vi "PH_PP_CurrentMeas.panel.vi"(0 "object ref":refnum<vi>, 5 "error in (no error)":errorcluster) -> (19 "error out":errorcluster)   [LabVIEW 2014, in "PH_PP_CurrentMeas.lvlib"]
doc: "This is just an example for a GUI thread.\n\nLicense Agreement for this software:\n\nCopyright (C)\nGesellschaft für Schwerionenforschung, GSI\nPlanckstr. 1\n64291 Darmstadt\nGermany\n\nContact: D.Beck@gsi.de \n\nThis program is free software; you can redistribute it and/or modify it under the terms of the GNU General Public License as published by the Free Software Foundation; either version 2 of the license, or (at your option) any later version.\n\nThis program is distributed in the hope that it will be useful, but WITHOUT ANYW ARRANTY; without even the implied warranty of MERCHANTABILITY or FITNESS FOR A PARTICULAR PURPOSE. See the GNU General License for more details (http://www.gnu.org).\n\nGesellschaft für Schwerionenforschung, GSI\nPlanckstr. 1, 64291 Darmstadt, Germany\nFor all questions and ideas contact: M.Richter@gsi.de, H.Brand@gsi.de or D.Beck@gsi.de.\nLast update: 18-DEC-2002"
uses:
  PH_PP_CurrentMeas.lvlib
  PH_Basics/PH_StatusHandler/PH_StatusHandler.GUI element.ctl
  PH_PP_CurrentMeas.CommandCluster.ctl
  CS_Core/CSObj/CSObj.lvlib
  PH_Basics/PH_Common/PH_Common.lvlib
  PH_Basics/PH_Class/PH_Class.lvlib
  PH_Basics/PH_PSDBWriter/PH_PSDBWriter.lvlib
  PH_Basics/PH_StatusHandler/PH_StatusHandler.lvlib
panel:
  in  "Start Task 3":bool
  in  "Start Task 2":bool
  in  "Start Task 1":bool
  out "Task FR and PPPA Bar":u32(colorbox) caption="Powermeter"
  out "Task PPMA FR and PPPA":u32(colorbox) caption="PPMA FR and PPPA"
  out "Task PPMA PU 3 ... 5 Bar":u32(colorbox) caption="Powermeter"
  out "Task PPMA PU 3 ... 5":u32(colorbox) caption="PPMA PU 3 ... 5"
  out "Task PPMA PU 1 ... 3 Bar":u32(colorbox) caption="Powermeter"
  out "Task PPMA PU 1 ... 3":u32(colorbox) caption="PPMA PU 1 ... 3"
  out "Sequencer State":string
  out "PSDB Status":u32(colorbox)=6618880 caption="PSDB"
  out "Status":T1 caption="Enabling State"
  in  "Exit":bool
  in  "stop":bool
  in  "Tab Control":T2(tab)
  out "PreAmp Data":waveform(dbl)[](graph) caption="Measurement data"
  out "Status 45mm":T1 caption="45mm"
  out "Status 19mm - 2":T1 caption="19mm - 2"
  out "Status 19mm - 1":T1 caption="19mm - 1"
  out "Data PU 1":waveform(dbl)[](graph) caption="Measurement data"
  out "Status PU1":T1 caption="Enabling State"
  out "Data PU 2":waveform(dbl)[](graph) caption="Measurement data"
  out "Status PU2":T1 caption="Enabling State"
  out "Data PU 3":waveform(dbl)[](graph) caption="Measurement data"
  out "Status PU3":T1 caption="Enabling State"
  out "Data PU 4":waveform(dbl)[](graph) caption="Measurement data"
  out "Status PU4":T1 caption="Enabling State"
  out "Data PU 5":waveform(dbl)[](graph) caption="Measurement data"
  out "Status PU5":T1 caption="Enabling State"
  out "Data PU FR":waveform(dbl)[](graph) caption="Measurement data"
  out "Status FR":T1 caption="Enabling State"
  out "Hardware Feedback":T4(array[cluster])
  # "PCS"
  # "3.40"
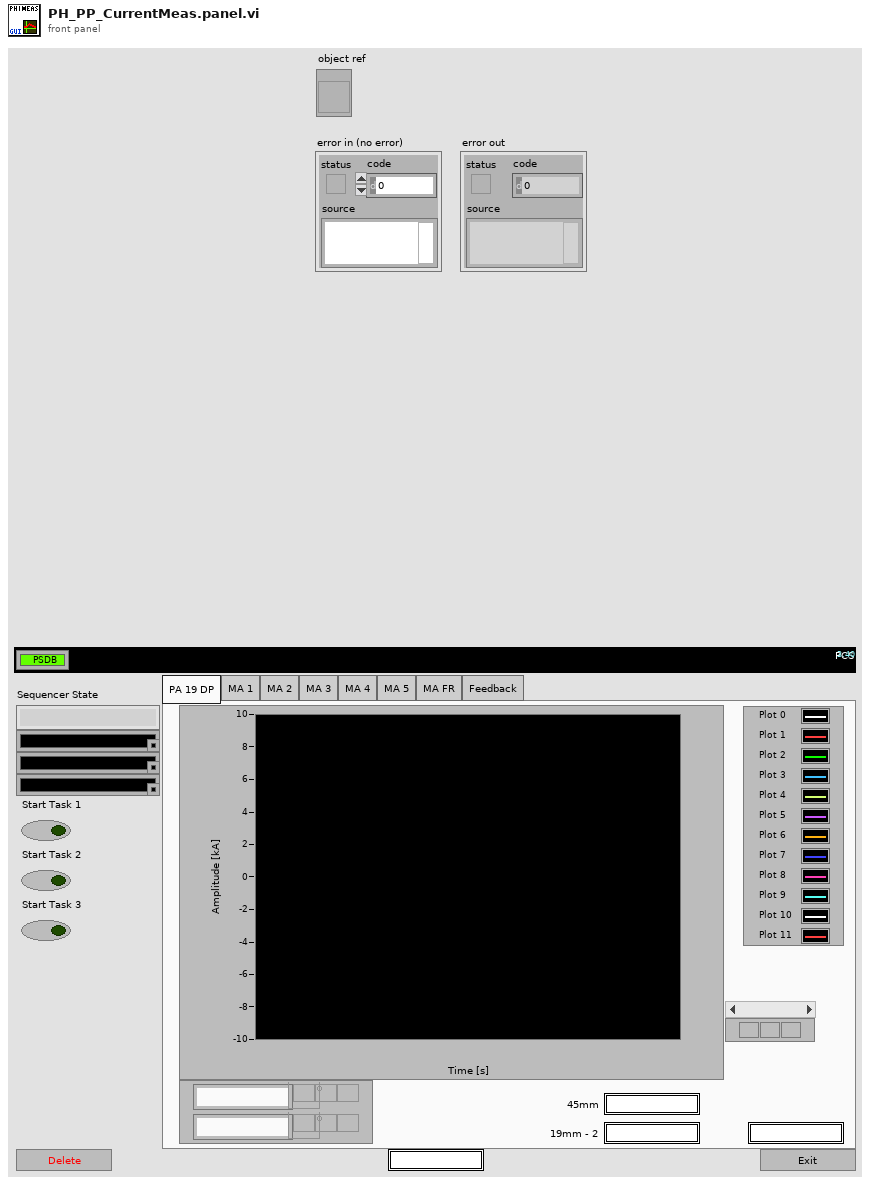
[diagram p1: front panel]
types:
  T1 = typedef "PH_StatusHandler.lvlib/PH_StatusHandler.GUI element.ctl" = u16
  T2 = enum32{"PA 19 DP", "MA 1", "MA 2", "MA 3", "MA 4", "MA 5", "MA FR", "Feedback"}
  T3 = typedef "PH_PP_CurrentMeas.lvlib/PH_PP_CurrentMeas.CommandCluster.ctl" = cluster{"Command":string, "Data":string, "error out":errorcluster}
  T4 = cluster{"Received Data Sets":T3[], "Driver Error":errorcluster, "Connection not established":bool, "Error unpacking the data":bool, "No Task defined":bool, "Not triggered yet":bool}[]
  T5 = typedef "PH_PP_CurrentMeas.lvlib/PH_PP_CurrentMeas.i attribute.ctl" = cluster{"Status":cluster{"GUI Ref Hardware Feedback":refnum<vi>, "Tab Control":refnum<vi>}, "PU 1":cluster{"Instance":string, "Status":T6, "Ref Status ":refnum<vi>, "Data":waveform(dbl)[], "Ref Data":refnum<vi>}, "PU 2":cluster{"Instance":string, "Status":T6, "Ref Status ":refnum<vi>, "Data":waveform(dbl)[], "Ref Data":refnum<vi>}, "PU 3":cluster{"Instance":string, "Status":T6, "Ref Status ":refnum<vi>, "Data":waveform(dbl)[], "Ref Data":refnum<vi>}, "PU 4":cluster{"Instance":string, "Status":T6, "Ref Status ":refnum<vi>, "Data":waveform(dbl)[], "Ref Data":refnum<vi>}, "PU 5":cluster{"Instance":string, "Status":T6, "Ref Status ":refnum<vi>, "Data":waveform(dbl)[], "Ref Data":refnum<vi>}, "FR":cluster{"Instance":string, "Status":T6, "Ref Status ":refnum<vi>, "Data":waveform(dbl)[], "Ref Data":refnum<vi>}, "PA - 19mm 1":cluster{"Instance":string, "Status":T6, "Ref Status ":refnum<vi>}, "PA - 19mm 2":cluster{"Instance":string, "Status":T6, "Ref Status ":refnum<vi>, "no link":bool}, "PA - 45mm":cluster{"Instance":string, "Status":T6, "Ref Status ":refnum<vi>, "no link":bool}, "PA Data":cluster{"Data":waveform(dbl)[], "Ref":refnum<vi>}, "Sequencer":cluster{"Instance":string, "SM State Ref":refnum<vi>}, "Tasks":cluster{"Port":u16, "connection ID":refnum<k5>, "Status":T6, "Ref":refnum<vi>, "Ref Bar":refnum<vi>, "Feedback":cluster{"Received Data Sets":T3[], "Driver Error":errorcluster, "Connection not established":bool, "Error unpacking the data":bool, "No Task defined":bool, "Not triggered yet":bool}, "Data":waveform(dbl)[], "Ref Teststart Task":refnum<vi>}[], "in use":cluster{"MA DP":bool, "FR and PA":bool}, "DAQ Server":string}
  T6 = typedef "PH_StatusHandler.lvlib/PH_StatusHandler.Status.ctl" = i16
  T7 = cluster{"Port":u16, "connection ID":refnum<k5>, "Status":T6, "Ref":refnum<vi>, "Ref Bar":refnum<vi>, "Feedback":cluster{"Received Data Sets":T3[], "Driver Error":errorcluster, "Connection not established":bool, "Error unpacking the data":bool, "No Task defined":bool, "Not triggered yet":bool}, "Data":waveform(dbl)[], "Ref Teststart Task":refnum<vi>}[]
  T8 = cluster{"Port":u16, "connection ID":refnum<k5>, "Status":T6, "Ref":refnum<vi>, "Ref Bar":refnum<vi>, "Feedback":cluster{"Received Data Sets":T3[], "Driver Error":errorcluster, "Connection not established":bool, "Error unpacking the data":bool, "No Task defined":bool, "Not triggered yet":bool}, "Data":waveform(dbl)[], "Ref Teststart Task":refnum<vi>}
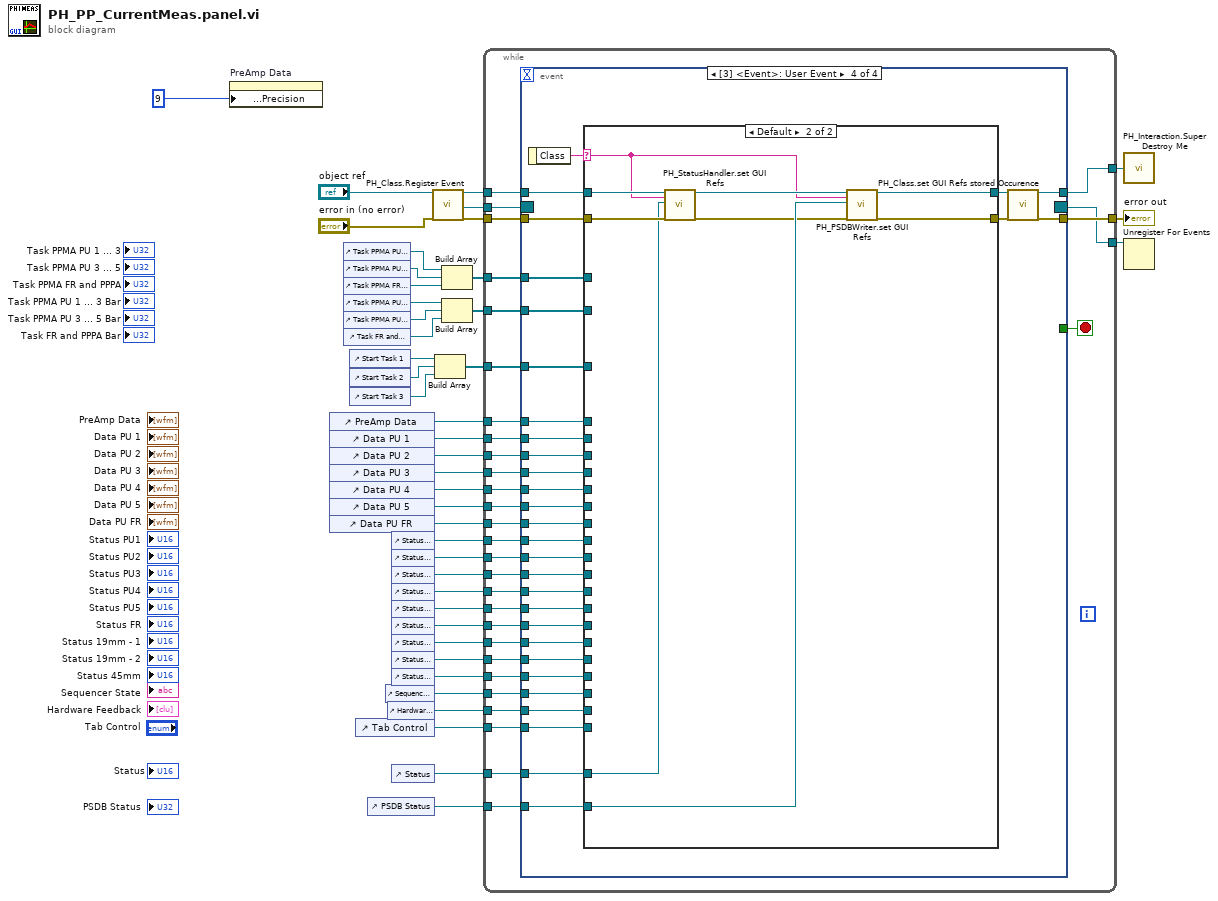
[diagram p0: block diagram]
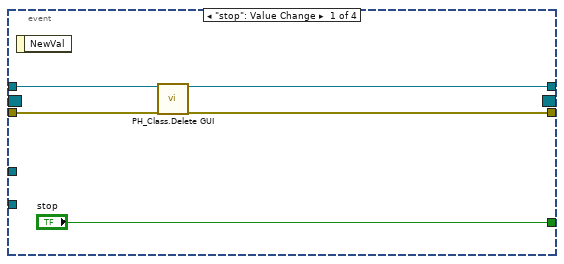
[diagram p2: hidden frame]
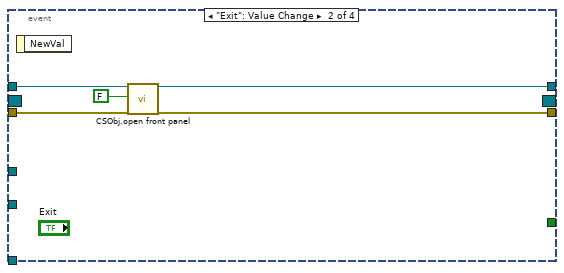
[diagram p3: hidden frame]
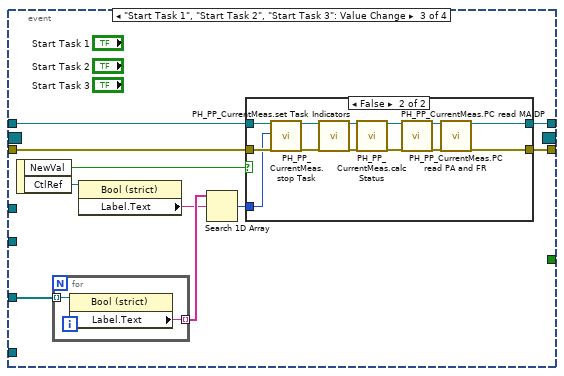
[diagram p4: hidden frame]
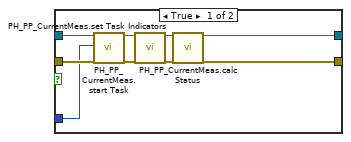
[diagram p5: hidden frame]
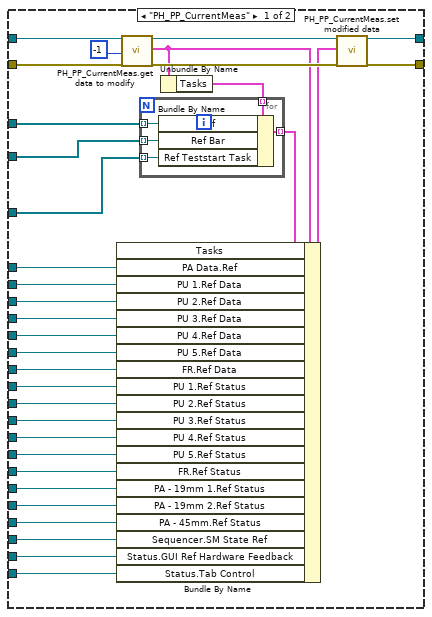
[diagram p6: hidden frame]
diagram:
  n1 = property on="PreAmp Data" class="WFGraph (strict)"("X Scale.Format & Precision:Precision"=u8 9) -> ()  [unwired: 2 in, 2 out]
  n2 = control-ref of="PreAmp Data"() -> (w20:refnum<vi>)
  n3 = control-ref of="Data PU 1"() -> (w19:refnum<vi>)
  n4 = control-ref of="Data PU 2"() -> (w18:refnum<vi>)
  n5 = control-ref of="Data PU 3"() -> (w17:refnum<vi>)
  n6 = control-ref of="Data PU 4"() -> (w16:refnum<vi>)
  n7 = control-ref of="Data PU 5"() -> (w15:refnum<vi>)
  n8 = control-ref of="Data PU FR"() -> (w14:refnum<vi>)
  n9 = control-ref of="Task PPMA PU 1 ... 3"() -> (w37:refnum<vi>)
  n10 = control-ref of="Task PPMA PU 3 ... 5"() -> (w38:refnum<vi>)
  n11 = control-ref of="Task PPMA FR and PPPA"() -> (w39:refnum<vi>)
  n12 = control-ref of="Task PPMA PU 1 ... 3 Bar"() -> (w36:refnum<vi>)
  n13 = control-ref of="Task PPMA PU 3 ... 5 Bar"() -> (w35:refnum<vi>)
  n14 = control-ref of="Task FR and PPPA Bar"() -> (w34:refnum<vi>)
  n15 = control-ref of="Start Task 1"() -> (w33:refnum<vi>)
  n16 = control-ref of="Start Task 2"() -> (w32:refnum<vi>)
  n17 = control-ref of="Start Task 3"() -> (w31:refnum<vi>)
  n18 = control-ref of="Tab Control"() -> (w11:refnum<vi>)
  n19 = control-ref of="PSDB Status"() -> (w25:refnum<vi>)
  n20 = control-ref of="Sequencer State"() -> (w13:refnum<vi>)
  n21 = control-ref of="Hardware Feedback"() -> (w12:refnum<vi>)
  n22 = control-ref of="Status PU1"() -> (w2:refnum<vi>)
  n23 = control-ref of="Status PU2"() -> (w3:refnum<vi>)
  n24 = control-ref of="Status PU3"() -> (w4:refnum<vi>)
  n25 = control-ref of="Status PU4"() -> (w5:refnum<vi>)
  n26 = control-ref of="Status PU5"() -> (w6:refnum<vi>)
  n27 = control-ref of="Status FR"() -> (w7:refnum<vi>)
  n28 = control-ref of="Status 19mm - 1"() -> (w8:refnum<vi>)
  n29 = control-ref of="Status 19mm - 2"() -> (w9:refnum<vi>)
  n30 = control-ref of="Status 45mm"() -> (w10:refnum<vi>)
  n31 = control-ref of="Status"() -> (w1:refnum<vi>)
  n32 = call "PH_Class.Register Event.vi"("i ref in"="object ref", "error in (no error)"="error in (no error)") -> ("i ref out"=w29:refnum<vi>, "Event Registration Refnum"=w27:refnum<event-registration>, "error out"=w28:errorcluster)  [unwired: 15 in]
  n33 = Build Array(w33, w32, w31) -> (w30:refnum<vi>[])
  n34 = Build Array(w37, w38, w39) -> (w24:refnum<vi>[])
  n35 = Build Array(w36, w35, w34) -> (w23:refnum<vi>[])
  n36 = while {
    tunnel: w29 -> [w72]
    tunnel: [w67] -> w41
    tunnel: w28 -> [w71]
    tunnel: [w70] -> w40
    tunnel: w30 -> [w69]
    tunnel: w27 -> [w68]
    tunnel: [w66] -> w26
    tunnel: w25 -> [w65]
    tunnel: w24 -> [w64]
    tunnel: w23 -> [w63]
    tunnel: w20 -> [w62]
    tunnel: w19 -> [w61]
    tunnel: w18 -> [w60]
    tunnel: w17 -> [w59]
    tunnel: w16 -> [w58]
    tunnel: w15 -> [w57]
    tunnel: w14 -> [w56]
    tunnel: w1 -> [w55]
    tunnel: w2 -> [w54]
    tunnel: w3 -> [w53]
    tunnel: w4 -> [w52]
    tunnel: w5 -> [w51]
    tunnel: w6 -> [w50]
    tunnel: w7 -> [w49]
    tunnel: w8 -> [w48]
    tunnel: w9 -> [w47]
    tunnel: w10 -> [w46]
    tunnel: w13 -> [w45]
    tunnel: w12 -> [w44]
    tunnel: w11 -> [w43]
    stop <- w73 stop-if-true
    n37 = event shown="[3] <Event>: User Event" {
      selector: w68 -> [_ _ _ _]
      dyn-events: [_ _ _ _] -> w66
      timeout: _ -> [_ _ _ _]
      tunnel: ["stop" _ _ _] -> w73
      tunnel: w72 -> [w76 w81 w91 w146]
      tunnel: [w75 w82 w92 w147] -> w70
      tunnel: w71 -> [w77 w83 w93 w145]
      tunnel: w69 -> [_ _ w88 w138]
      tunnel: [w74 w79 w84 w148] -> w67
      tunnel: w65 -> [_ _ _ w142]
      tunnel: w64 -> [_ _ _ w140]
      tunnel: w63 -> [_ _ _ w139]
      tunnel: w62 -> [_ _ _ w137]
      tunnel: w61 -> [_ _ _ w136]
      tunnel: w60 -> [_ _ _ w135]
      tunnel: w59 -> [_ _ _ w134]
      tunnel: w58 -> [_ _ _ w133]
      tunnel: w57 -> [_ _ _ w132]
      tunnel: w56 -> [_ _ _ w131]
      tunnel: w55 -> [_ _ _ w130]
      tunnel: w54 -> [_ _ _ w129]
      tunnel: w53 -> [_ _ _ w128]
      tunnel: w52 -> [_ _ _ w127]
      tunnel: w51 -> [_ _ _ w126]
      tunnel: w50 -> [_ _ _ w125]
      tunnel: w49 -> [_ _ _ w124]
      tunnel: w48 -> [_ _ _ w123]
      tunnel: w47 -> [_ _ _ w122]
      tunnel: w46 -> [_ _ _ w121]
      tunnel: w45 -> [_ _ _ w120]
      tunnel: w44 -> [_ _ _ w119]
      tunnel: w43 -> [_ _ _ w118]
      event "stop": Value Change {
        n38 = event-data() -> ()  [unwired: 1 in, 1 out]
        n39 = call "PH_Class.Delete GUI.vi"("VI in"=w76, "error in (no error)"=w77) -> ("VI out"=w74:refnum<vi>, "error out"=w75:errorcluster)  [unwired: 16 in]
      }
      event "Exit": Value Change {
        n40 = event-data() -> ()  [unwired: 1 in, 1 out]
        n41 = call "CSObj.open front panel.vi"("i ref in"=w81, "frontPanelOpen"=FALSE ("front panel open"), "error in (no error)"=w83) -> ("i ref out"=w79:refnum<vi>, "error out"=w82:errorcluster)  [unwired: 15 in]
      }
      event "Start Task 1", "Start Task 2", "Start Task 3": Value Change {
        n42 = event-data() -> ("NewVal"=w90:bool, "CtlRef"=w89:refnum<vi>)  [unwired: 1 in]
        n43 = for {
          tunnel: w88 -> [w95] mode=indexing
          tunnel: [w94] -> w87 mode=indexing
          n44 = property class="Bool (strict)"(reference=w95) -> ("Label.Text"=w94:string)  [unwired: 1 in, 2 out]
        }
        n45 = property class="Bool (strict)"(reference=w89) -> ("Label.Text"=w86:string)  [unwired: 1 in, 2 out]
        n46 = Search 1D Array(1D array=w87, element=w86) -> (index of element=w85:i32)  [unwired: 1 in]
        n47 = case shown="False" w90 {
          tunnel: w93 -> [w104 w117]
          tunnel: [w97 w106] -> w92
          tunnel: w91 -> [w103 w116]
          tunnel: w85 -> [w102 w115]
          tunnel: [w96 w105] -> w84
          frame True {
            n48 = call "PH_PP_CurrentMeas.start Task.vi"("i ref in"=w103, "Task #"=w102, "error in (no error)"=w104) -> ("i ref out"=w98:refnum<vi>, "error out"=w99:errorcluster)  [unwired: 15 in]
            n49 = call "PH_PP_CurrentMeas.set Task Indicators.vi"("i ref in"=w98, "error in (no error)"=w99) -> ("i ref out"=w101:refnum<vi>, "error out"=w100:errorcluster)  [unwired: 16 in]
            n50 = call "PH_PP_CurrentMeas.calc Status.vi"("i ref in"=w101, "error in (no error)"=w100) -> ("i ref out"=w96:refnum<vi>, "error out"=w97:errorcluster)  [unwired: 16 in]
          }
          frame False {
            n51 = call "PH_PP_CurrentMeas.stop Task.vi"("i ref in"=w116, "Task #"=w115, "error in (no error)"=w117) -> ("i ref out"=w111:refnum<vi>, "error out"=w112:errorcluster)  [unwired: 15 in]
            n52 = call "PH_PP_CurrentMeas.set Task Indicators.vi"("i ref in"=w111, "error in (no error)"=w112) -> ("i ref out"=w114:refnum<vi>, "error out"=w113:errorcluster)  [unwired: 16 in]
            n53 = call "PH_PP_CurrentMeas.calc Status.vi"("i ref in"=w114, "error in (no error)"=w113) -> ("i ref out"=w107:refnum<vi>, "error out"=w108:errorcluster)  [unwired: 16 in]
            n54 = call "PH_PP_CurrentMeas.PC read MA DP.vi"("i ref in"=w107, "error in (no error)"=w108) -> ("i ref out"=w109:refnum<vi>, "error out"=w110:errorcluster)  [unwired: 16 in]
            n55 = call "PH_PP_CurrentMeas.PC read PA and FR.vi"("i ref in"=w109, "error in (no error)"=w110) -> ("i ref out"=w105:refnum<vi>, "error out"=w106:errorcluster)  [unwired: 16 in]
          }
        }
      }
      event User Event {
        n56 = event-data() -> ("Class"=w141:string)  [unwired: 1 in]
        n57 = case shown="Default" w141 {
          selector: w141 -> [_ w188]
          tunnel: w146 -> [w175 w190]
          tunnel: w145 -> [w173 w195]
          tunnel: [w174 w194] -> w144
          tunnel: [w172 w193] -> w143
          tunnel: w142 -> [_ w192]
          tunnel: w140 -> [w170 _]
          tunnel: w139 -> [w169 _]
          tunnel: w138 -> [w168 _]
          tunnel: w137 -> [w167 _]
          tunnel: w136 -> [w166 _]
          tunnel: w135 -> [w165 _]
          tunnel: w134 -> [w164 _]
          tunnel: w133 -> [w163 _]
          tunnel: w132 -> [w162 _]
          tunnel: w131 -> [w161 _]
          tunnel: w130 -> [_ w187]
          tunnel: w129 -> [w160 _]
          tunnel: w128 -> [w159 _]
          tunnel: w127 -> [w158 _]
          tunnel: w126 -> [w157 _]
          tunnel: w125 -> [w156 _]
          tunnel: w124 -> [w155 _]
          tunnel: w123 -> [w154 _]
          tunnel: w122 -> [w153 _]
          tunnel: w121 -> [w152 _]
          tunnel: w120 -> [w151 _]
          tunnel: w119 -> [w150 _]
          tunnel: w118 -> [w149 _]
          frame "PH_PP_CurrentMeas" {
            n58 = call "PH_PP_CurrentMeas.get data to modify.vi"("i ref in"=w175, "ms timeout (10000)"=-1, "error in (no error)"=w173) -> ("i ref out"=w181:refnum<vi>, "i attribute"=w178:T5, "error out"=w180:errorcluster)  [unwired: 13 in, 1 out]
            n59 = Unbundle By Name(w178) -> ("Tasks"=w177:T7)
            n60 = for {
              tunnel: w177 -> [w186] mode=indexing
              tunnel: [w185] -> w176 mode=indexing
              tunnel: w170 -> [w184] mode=indexing
              tunnel: w169 -> [w183] mode=indexing
              tunnel: w168 -> [w182] mode=indexing
              n61 = Bundle By Name(cluster=w186, "Ref"=w184, "Ref Bar"=w183, "Ref Teststart Task"=w182) -> (w185:T8)
            }
            n62 = Bundle By Name(cluster=w178, "Tasks"=w176, "PA Data.Ref"=w167, "PU 1.Ref Data"=w166, "PU 2.Ref Data"=w165, "PU 3.Ref Data"=w164, "PU 4.Ref Data"=w163, "PU 5.Ref Data"=w162, "FR.Ref Data"=w161, "PU 1.Ref Status"=w160, "PU 2.Ref Status"=w159, "PU 3.Ref Status"=w158, "PU 4.Ref Status"=w157, "PU 5.Ref Status"=w156, "FR.Ref Status"=w155, "PA - 19mm 1.Ref Status"=w154, "PA - 19mm 2.Ref Status"=w153, "PA - 45mm.Ref Status"=w152, "Sequencer.SM State Ref"=w151, "Status.GUI Ref Hardware Feedback"=w150, "Status.Tab Control"=w149) -> (w179:T5)
            n63 = call "PH_PP_CurrentMeas.set modified data.vi"("i ref in"=w181, "i attribute"=w179, "error in (no error)"=w180) -> ("i ref out"=w174:refnum<vi>, "error out"=w172:errorcluster)  [unwired: 15 in]
          }
          frame Default {
            n64 = call "PH_StatusHandler.set GUI Refs.vi"("i ref in"=w190, "Class"=w188, "GUI Ref"=w187, "error in (no error)"=w195) -> ("i ref out"=w189:refnum<vi>, "error out"=w191:errorcluster)  [unwired: 14 in]
            n65 = call "PH_PSDBWriter.set GUI Refs.vi"("i ref in"=w189, "Class"=w188, "Ref PSDB Status"=w192, "error in"=w191) -> ("i ref out"=w194:refnum<vi>, "error out"=w193:errorcluster)  [unwired: 14 in]
          }
        }
        n66 = call "PH_Class.set GUI Refs stored Occurence.vi"("i ref in"=w144, "error in (no error)"=w143) -> ("i ref out"=w148:refnum<vi>, "error out"=w147:errorcluster)  [unwired: 16 in]
      }
    }
  }
  "error out" <- w40
  n67 = call "PH_Interaction.Super Destroy Me.vi"("i ref out"=w41) -> ()
  n68 = Unregister For Events(event registration refnum=w26) -> ()  [unwired: 1 in, 1 out]
